vi "Assignment W3.vi"() -> ()   [LabVIEW 2022 SP3]
panel:
  out "?":string
  in  "Choose your product's brand":enum16{"Samsung", "LG", "Bosch"}(ring)
  in  "Stop Looping":bool
  out "Product's warranty":dbl
  out "Product's power":dbl
  out "Product's price":dbl
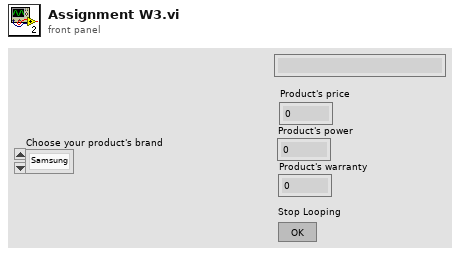
[diagram p1: front panel]
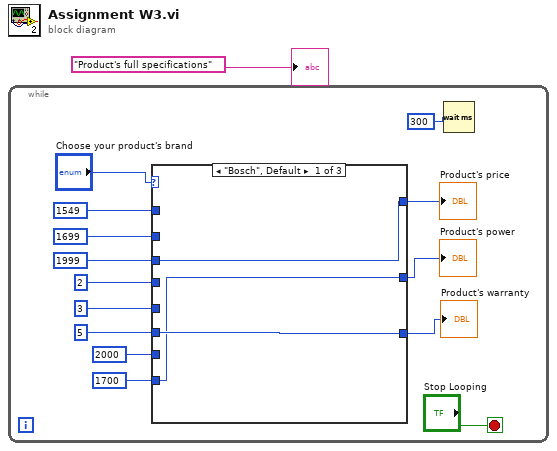
[diagram p0: block diagram]
diagram:
  n1 = while {
    stop <- "Stop Looping" stop-if-true
    n2 = case shown="\"Bosch\", Default" "Choose your product's brand" {
      tunnel: 1699 -> [_ _ w24]
      tunnel: 3 -> [_ _ w22]
      tunnel: 5 -> [w17 _ _]
      tunnel: 2000 -> [_ w19 w23]
      tunnel: 1700 -> [w16 _ _]
      tunnel: 1549 -> [_ w21 _]
      tunnel: 1999 -> [w18 _ _]
      tunnel: [w18 w21 w24] -> w8
      tunnel: [w17 w20 w22] -> w7
      tunnel: [w16 w19 w23] -> w6
      tunnel: 2 -> [_ w20 _]
      frame "Bosch", Default {
      }
      frame "Samsung" {
      }
      frame "LG" {
      }
    }
    "Product's price" <- w8
    "Product's power" <- w6
    "Product's warranty" <- w7
    n3 = Wait (ms)(milliseconds to wait=300) -> ()  [unwired: 1 out]
  }
  "?" <- "Product's full specifications"
